vi "ResultsHandlerTCP.vi"(8 "error":errorcluster, 9 "JSON-request":string="{\"jsonrpc\":\"2.0\",\"method\":\"com.attocube.amc.control.getActorType\",\"params\":[0],\"id\":\"1\",\"api\":2}", 10 "JSON-response":string, 11 "results_cluster":refnum<vi>[](array[refnum])) -> (0 "error":errorcluster)   [LabVIEW 2016]
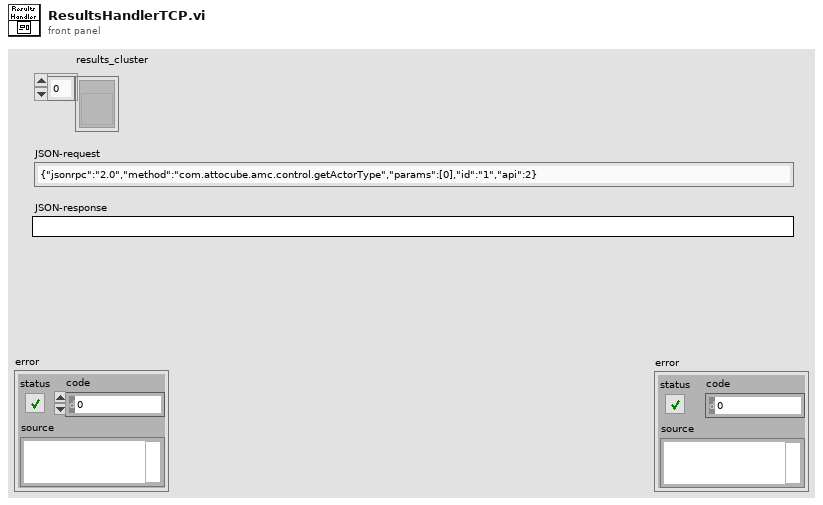
[diagram p1: front panel]
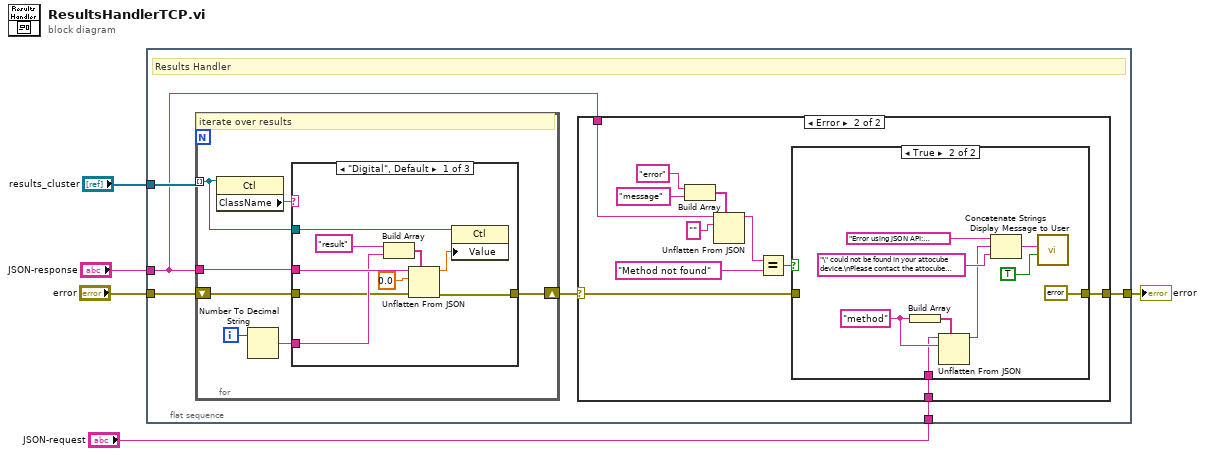
[diagram p0: block diagram]
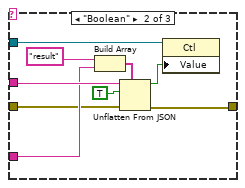
[diagram p4: hidden frame]
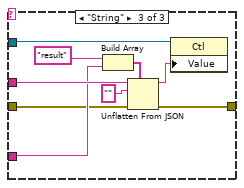
[diagram p5: hidden frame]
diagram:
  n1 = flat-sequence {
    tunnel: "results_cluster" -> [w11]
    tunnel: "JSON-response" -> [w8]
    tunnel: [w7] -> w3
    tunnel: "error" -> [w10]
    tunnel: "JSON-request" -> [w6]
    frame #0 {
      # "Results Handler"
      n2 = for {
        tunnel: w8 -> [w40]
        tunnel: w11 -> [w36] mode=indexing
        shift-right: [w34] -> w9
        shift-left: w10 -> [w35]
        i -> [w39]
        # "iterate over results"
        n3 = property class="Ctl"(reference=w36) -> ("ClassName"=w37:string)  [unwired: 1 in, 2 out]
        n4 = Number To Decimal String(number=w39) -> (decimal integer string=w38:string)  [unwired: 1 in]
        n5 = case shown="\"Digital\", Default" w37 {
          tunnel: w40 -> [w44 w54 w62]
          tunnel: w38 -> [w43 w53 w61]
          tunnel: w36 -> [w45 w52 w63]
          tunnel: [w41 w50 w60] -> w34
          tunnel: w35 -> [w42 w51 w59]
          frame "Digital", Default {
            n6 = Build Array("result", w43) -> (w47:string[])
            n7 = Unflatten From JSON(path=w47, JSON string=w44, type and defaults=0.0, error in (no error)=w42) -> (value=w46:dbl, error out=w41:errorcluster)  [unwired: 3 in]
            n8 = property class="Ctl"(reference=w45, "Value"=w46) -> ()  [unwired: 1 in, 2 out]
          }
          frame "Boolean" {
            n9 = Build Array("result", w53) -> (w56:string[])
            n10 = Unflatten From JSON(path=w56, JSON string=w54, type and defaults=TRUE, error in (no error)=w51) -> (value=w55:bool, error out=w50:errorcluster)  [unwired: 3 in]
            n11 = property class="Ctl"(reference=w52, "Value"=w55) -> ()  [unwired: 1 in, 2 out]
          }
          frame "String" {
            n12 = Build Array("result", w61) -> (w65:string[])
            n13 = Unflatten From JSON(path=w65, JSON string=w62, type and defaults="", error in (no error)=w59) -> (value=w64:string, error out=w60:errorcluster)  [unwired: 3 in]
            n14 = property class="Ctl"(reference=w63, "Value"=w64) -> ()  [unwired: 1 in, 2 out]
          }
        }
      }
      n15 = case shown="Error" w9 {
        selector: w9 -> [w12 w15]
        tunnel: w8 -> [_ w17]
        tunnel: [w12 w14] -> w7
        tunnel: w6 -> [_ w13]
        frame No Error {
        }
        frame Error {
          n16 = Build Array("error", "message" ("element")) -> (w22:string[])
          n17 = Unflatten From JSON(path=w22, JSON string=w17, type and defaults="") -> (value=w19:string)  [unwired: 4 in, 1 out]
          n18 = Equal?(x=w19, y="Method not found") -> (x = y?=w16:bool)
          n19 = case shown="True" w16 {
            tunnel: w15 -> [w24 _]
            tunnel: [w24 errorcluster {"status"=TRUE, "code"=-32601, "source"="TCP Handler: \"Method not found\" Error within attocube device"} ("error out 3")] -> w14
            tunnel: w13 -> [_ w27]
            frame False {
            }
            frame True {
              w28 = "method"
              n20 = Build Array(w28) -> (w29:string[])
              n21 = Unflatten From JSON(path=w29, JSON string=w27, type and defaults=w28) -> (value=w31:string)  [unwired: 4 in, 1 out]
              n22 = Concatenate Strings("Error using JSON API: Method \"", w31, "\" could not be found in your attocube device.\nPlease contact the attocube support team.") -> (w26:string)
              n23 = call "Display Message to User"("Enable"=TRUE, "Message"=w26) -> ()  [unwired: 8 in, 2 out]
            }
          }
        }
      }
    }
  }
  "error" <- w3
